vi "Editor.vi"() -> ()   [LabVIEW 2010]
uses:
  Components/Components.lvlib
panel:
  out "Current File":path caption="selected path"
  in  "Save As":bool
  in  "Refresh":bool
  in  "Update":bool
  out "Frame Size":u16=8
  in  "Frames":cluster{"Time":u32, "Powers":i16[]}[](array[cluster]) caption="Frame"
  out "Header":string
  in  "Number Of Motors":u8=2
  in  "Storage Size":enum8{"I8", "I16"}(ring)=enum."I16"
  out "File":refnum<file>
  in  "Writing?":bool
  in  "Cancel":bool
  in  "Open":bool
  in  "New":bool
  out "Binary Out":string
  in  "Save":bool
  # "4BC Editor"
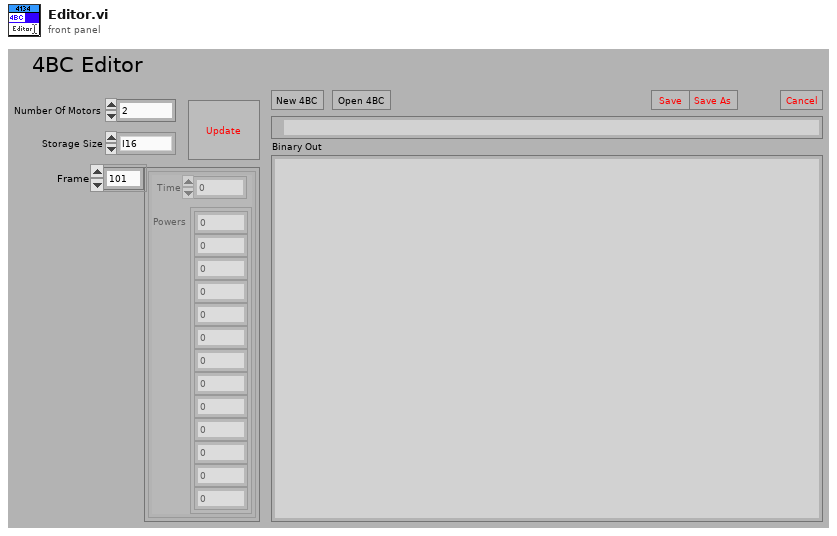
[diagram p1: front panel]
types:
  T1 = enum16{"open", "replace", "create", "open or create", "replace or create", "replace or create with confirmation"}
  T2 = enum16{"big-endian, network order", "native, host order", "little-endian"}
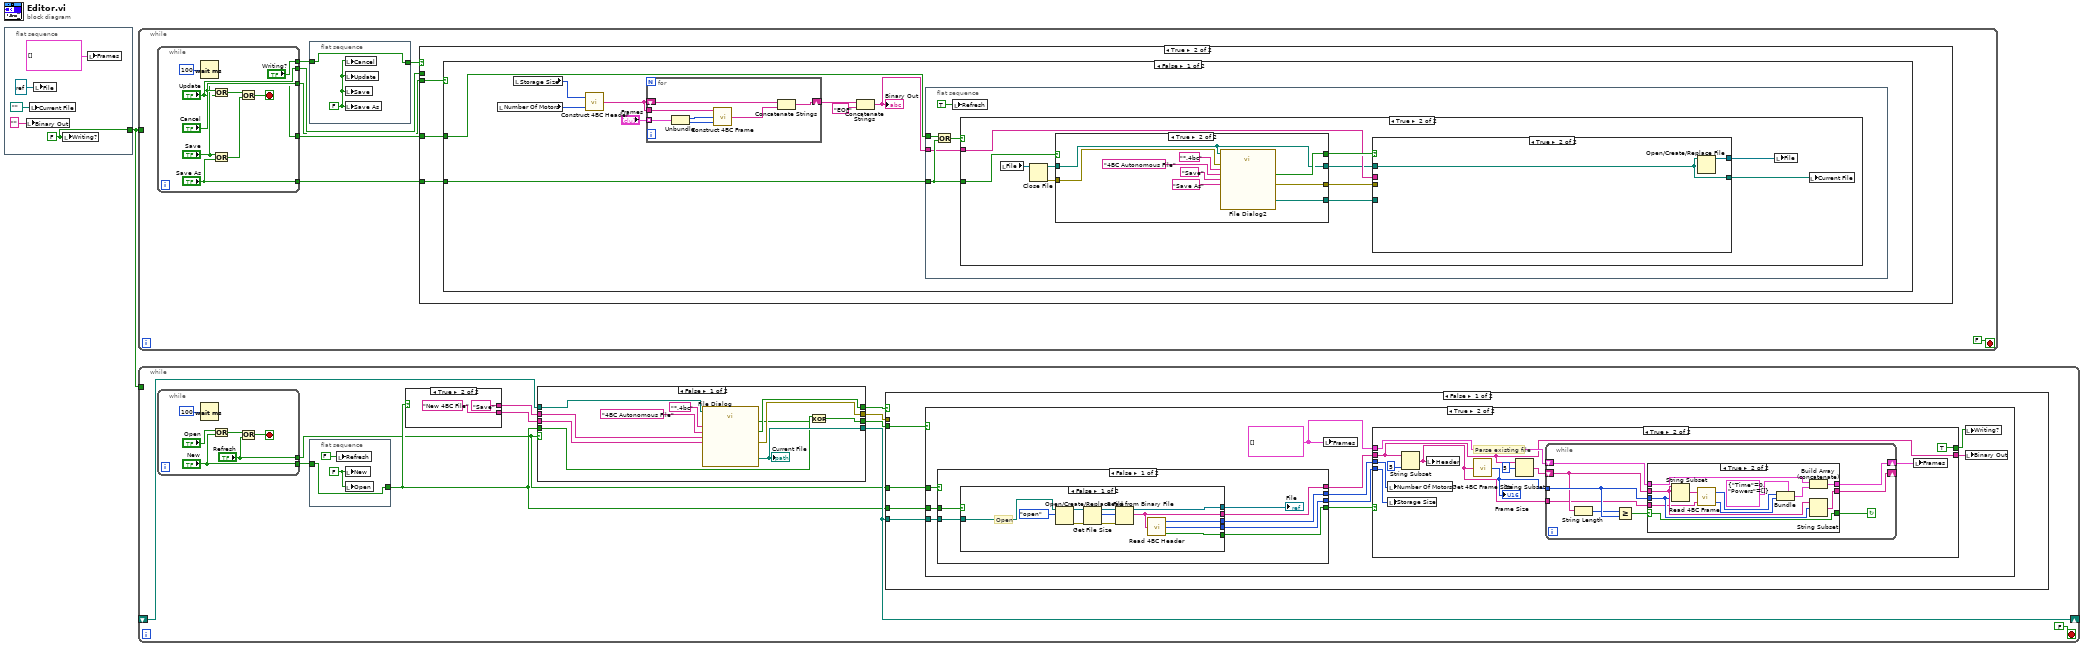
[diagram p0: block diagram]
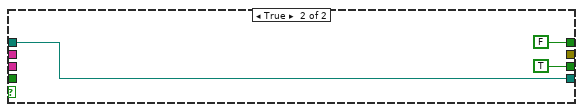
[diagram p2: hidden frame]
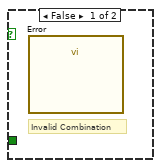
[diagram p3: hidden frame]
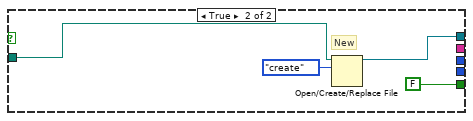
[diagram p4: hidden frame]
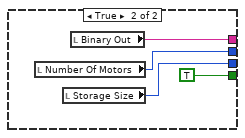
[diagram p5: hidden frame]
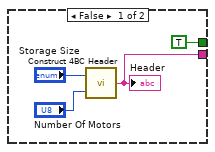
[diagram p6: hidden frame]
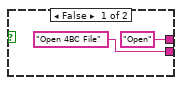
[diagram p9: hidden frame]
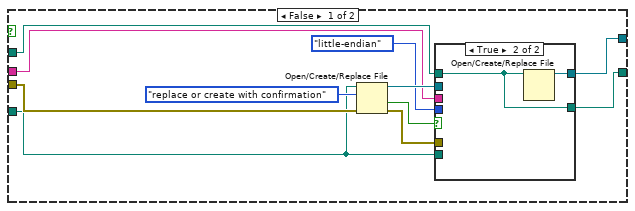
[diagram p12: hidden frame]
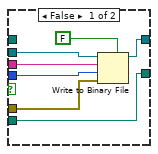
[diagram p13: hidden frame]
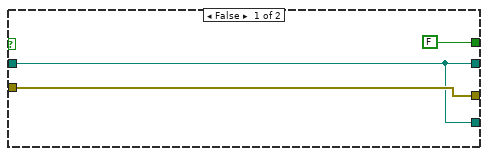
[diagram p14: hidden frame]
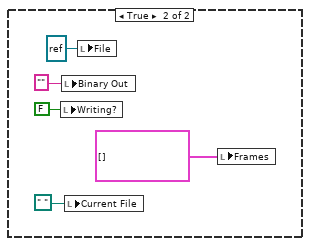
[diagram p15: hidden frame]
diagram:
  n1 = flat-sequence {
    tunnel: [w6] -> w1
    frame #0 {
      w6 = FALSE ("Writing?")
      n2 = local write "Binary Out"("" ("Binary Out")) -> ()
      n3 = local write "Current File"(path "" ("Current File")) -> ()
      n4 = local write "File"(refnum<file> refnum ("File")) -> ()
      n5 = local write "Writing?"(w6) -> ()
      n6 = local write "Frames"(cluster{"Time":u32, "Powers":i16[]}[] [] ("Frames")) -> ()
    }
  }
  n7 = while {
    tunnel: w1 -> [_]
    stop <- FALSE stop-if-true
    n8 = while {
      tunnel: ["Writing?"] -> w10
      tunnel: ["Save"] -> w11
      tunnel: ["Update"] -> w12
      tunnel: ["Cancel"] -> w8
      tunnel: ["Save As"] -> w7
      stop <- w97 stop-if-true
      n9 = Wait (ms)(milliseconds to wait=u32 100) -> ()  [unwired: 1 out]
      n10 = Or(x="Cancel", y="Update") -> (x .or. y?=w93:bool)
      n11 = Or(x="Save", y="Save As") -> (x .or. y?=w94:bool)
      n12 = Or(x=w93, y=w94) -> (x .or. y?=w97:bool)
    }
    n13 = flat-sequence {
      tunnel: w10 -> [w15]
      tunnel: [w15] -> w9
      frame #0 {
        w14 = FALSE ("Cancel")
        n14 = local write "Cancel"(w14) -> ()
        n15 = local write "Update"(w14) -> ()
        n16 = local write "Save"(w14) -> ()
        n17 = local write "Save As"(w14) -> ()
      }
    }
    n18 = case shown="True" w9 {
      tunnel: w12 -> [_ _]
      tunnel: w11 -> [_ w17]
      tunnel: w8 -> [_ w18]
      tunnel: w7 -> [_ w16]
      frame False {
      }
      frame True {
        n19 = case shown="False" w18 {
          tunnel: w17 -> [w19 _]
          tunnel: w16 -> [w20 _]
          frame False {
            n20 = local read "Number Of Motors"() -> (w26:u8)
            n21 = local read "Storage Size"() -> (w27:enum8{"I8", "I16"})
            n22 = call "Construct 4BC Header.vi"("Number Of Motors"=w26, "Storage Size"=w27) -> ("Header"=w24:string)
            n23 = for {
              shift-right: [w78] -> w23
              shift-left: w24 -> [w79]
              tunnel: "Frames" -> [w84] mode=indexing
              tunnel: w24 -> [w81]
              n24 = Unbundle(w84) -> ("Time"=w83:u32, "Powers"=w82:i16[])
              n25 = call "Construct 4BC Frame.vi"("Array"=w82, "Time"=w83, "Header"=w81) -> ("Frame"=w80:string)  [unwired: 1 in]
              n26 = Concatenate Strings(w79, w80) -> (w78:string)
            }
            n27 = Concatenate Strings(w23, "EOF" ("string")) -> (w21:string)
            "Binary Out" <- w21
            n28 = flat-sequence {
              tunnel: w21 -> [w28]
              tunnel: w20 -> [w30]
              tunnel: w19 -> [w29]
              frame #0 {
                n29 = Or(x=w29, y=w30) -> (x .or. y?=w31:bool)
                n30 = local write "Refresh"(TRUE ("Refresh")) -> ()
                n31 = case shown="True" w31 {
                  tunnel: w30 -> [_ w42]
                  tunnel: w28 -> [_ w36]
                  frame False {
                  }
                  frame True {
                    n32 = local read "File"() -> (w43:refnum<file>)
                    n33 = Close File(refnum=w43) -> (path=w41:path, error out=w40:errorcluster)  [unwired: 1 in]
                    n34 = case shown="True" w42 {
                      tunnel: w41 -> [w66 w69]
                      tunnel: w40 -> [w68 w77]
                      tunnel: [w68 w72] -> w39
                      tunnel: [w66 w71] -> w38
                      tunnel: [FALSE ("cancelled") w70] -> w37
                      tunnel: [w66 w69] -> w35
                      frame False {
                      }
                      frame True {
                        n35 = call "File Dialog2"("start path"=w69, "prompt"="Save As", "button label"="Save", "error in"=w77, "pattern (all files)"="*.4bc", "pattern label"="4BC Autonomous File") -> ("selected path"=w71:path, "cancelled"=w70:bool, "error out"=w72:errorcluster)  [unwired: 6 in, 1 out]
                      }
                    }
                    n36 = case shown="True" w37 {
                      tunnel: w39 -> [w53 _]
                      tunnel: w38 -> [w47 _]
                      tunnel: w36 -> [w51 _]
                      tunnel: w35 -> [w46 w64]
                      tunnel: [w45 w65] -> w34
                      tunnel: [w44 w64] -> w33
                      frame False {
                        n37 = Open/Create/Replace File(file path (use dialog)=w47, error in=w53, operation (0:open)=T1."replace or create with confirmation") -> (refnum out=w54:refnum<file>, cancelled=w48:bool, error out=w49:errorcluster)  [unwired: 3 in]
                        n38 = case shown="True" w48 {
                          tunnel: w54 -> [w61 _]
                          tunnel: T2."little-endian" ("byte order (0:big-endian, network order)") -> [w59 _]
                          tunnel: w51 -> [w58 _]
                          tunnel: w49 -> [w57 _]
                          tunnel: w47 -> [w55 _]
                          tunnel: [w56 w63] -> w45
                          tunnel: [w55 w62] -> w44
                          tunnel: w46 -> [_ w62]
                          frame False {
                            n39 = Write to Binary File(file (use dialog)=w61, data=w58, error in=w57, 5:FALSE ("prepend array or string size? (T)"), 9:w59) -> (refnum out=w56:refnum<file>)  [unwired: 1 in, 2 out]
                          }
                          frame True {
                            n40 = Open/Create/Replace File(file path (use dialog)=w62) -> (refnum out=w63:refnum<file>)  [unwired: 5 in, 2 out]
                          }
                        }
                      }
                      frame True {
                        n41 = Open/Create/Replace File(file path (use dialog)=w64) -> (refnum out=w65:refnum<file>)  [unwired: 5 in, 2 out]
                      }
                    }
                    n42 = local write "File"(w34) -> ()
                    n43 = local write "Current File"(w33) -> ()
                  }
                }
              }
            }
          }
          frame True {
            n44 = local write "Writing?"(FALSE ("Writing?")) -> ()
            n45 = local write "Binary Out"("" ("Binary Out")) -> ()
            n46 = local write "Current File"(path " " ("Current File")) -> ()
            n47 = local write "File"(refnum<file> refnum ("File")) -> ()
            n48 = local write "Frames"(cluster{"Time":u32, "Powers":i16[]}[] [] ("Frames")) -> ()
          }
        }
      }
    }
  }
  n49 = while {
    shift-right: [w104] -> _
    shift-left: _ -> [w106]
    tunnel: w1 -> [_]
    stop <- FALSE stop-if-true
    n50 = while {
      tunnel: ["New"] -> w105
      tunnel: ["Refresh"] -> w99
      stop <- w212 stop-if-true
      n51 = Wait (ms)(milliseconds to wait=u32 100) -> ()  [unwired: 1 out]
      n52 = Or(x="Open", y="New") -> (x .or. y?=w213:bool)
      n53 = Or(x=w213, y="Refresh") -> (x .or. y?=w212:bool)
    }
    n54 = flat-sequence {
      tunnel: w105 -> [w205]
      tunnel: [w205] -> w100
      frame #0 {
        w206 = FALSE ("New")
        n55 = local write "Refresh"(FALSE ("Refresh")) -> ()
        n56 = local write "New"(w206) -> ()
        n57 = local write "Open"(w206) -> ()
      }
    }
    n58 = case shown="True" w100 {
      tunnel: ["Open" "Save"] -> w107
      tunnel: ["Open 4BC File" "New 4BC File"] -> w108
      frame False {
      }
      frame True {
      }
    }
    n59 = case shown="False" w99 {
      tunnel: w108 -> [w118 _]
      tunnel: w107 -> [w117 _]
      tunnel: w106 -> [w116 w121]
      tunnel: [w115 w121] -> w104
      tunnel: [w114 FALSE ("cancelled")] -> w103
      tunnel: [w110 TRUE] -> w101
      tunnel: [w113 _] -> w102
      tunnel: w100 -> [w112 _]
      frame False {
        n60 = call "File Dialog"("start path"=w116, "prompt"=w118, "button label"=w117, "pattern (all files)"="*.4bc", "pattern label"="4BC Autonomous File") -> ("selected path"=w115:path, "exists"=w111:bool, "cancelled"=w114:bool, "error out"=w113:errorcluster)  [unwired: 7 in]
        "Current File" <- w115
        n61 = Exclusive Or(1:w111, 2:w112) -> (0:w110:bool)
      }
      frame True {
      }
    }
    n62 = case shown="False" w103 {
      tunnel: w104 -> [w125 _]
      tunnel: w101 -> [w127 _]
      tunnel: w100 -> [w126 _]
      tunnel: w102 -> [_ _]
      tunnel: w99 -> [w124 _]
      frame False {
        n63 = case shown="True" w127 {
          tunnel: w126 -> [_ w137]
          tunnel: w125 -> [_ w136]
          tunnel: w124 -> [_ w128]
          frame False {
            # "Invalid Combination"
            n64 = call "Error"() -> ()  [unwired: 18 in, 2 out]
          }
          frame True {
            w130 = cluster{"Time":u32, "Powers":i16[]}[] [] ("Frames 2")
            n65 = case shown="False" w128 {
              tunnel: w137 -> [w144 _]
              tunnel: w136 -> [w143 _]
              tunnel: [w141 TRUE ("Valid?")] -> w135
              tunnel: [w140 w163] -> w134
              tunnel: [w139 w161] -> w133
              tunnel: [w138 w162] -> w132
              frame False {
                n66 = case shown="False" w144 {
                  tunnel: w143 -> [w155 w159]
                  tunnel: [w156 w158] -> w142
                  tunnel: [w145 _] -> w140
                  tunnel: [w148 FALSE] -> w141
                  tunnel: [w147 _] -> w139
                  tunnel: [w146 _] -> w138
                  frame False {
                    # "Open"
                    n67 = Open/Create/Replace File(file path (use dialog)=w155, operation (0:open)=T1."open") -> (refnum out=w152:refnum<file>, error out=w150:errorcluster)  [unwired: 4 in, 1 out]
                    n68 = Get File Size(file=w152, error in=w150) -> (refnum out=w151:refnum<file>, size (in bytes)=w153:i64, 0:w149:errorcluster)
                    n69 = Read from Binary File(8:w149, 10:w153, 11:w151) -> (2:w145:string, 3:w156:refnum<file>)  [unwired: 3 in, 2 out]
                    n70 = call "Read 4BC Header.vi"("Header"=w145) -> ("Valid?"=w148:bool, "Storage Size"=w147:enum8{"I8", "I16"}, "Number Of Motors"=w146:u8)
                  }
                  frame True {
                    # "New"
                    n71 = Open/Create/Replace File(file path (use dialog)=w159, operation (0:open)=T1."create") -> (refnum out=w158:refnum<file>)  [unwired: 4 in, 2 out]
                  }
                }
                "File" <- w142
              }
              frame True {
                n72 = local read "Number Of Motors"() -> (w162:u8)
                n73 = local read "Storage Size"() -> (w161:enum8{"I8", "I16"})
                n74 = local read "Binary Out"() -> (w163:string)
              }
            }
            n75 = local write "Frames"(w130) -> ()
            n76 = case shown="True" w135 {
              tunnel: w134 -> [_ w171]
              tunnel: w133 -> [_ w179]
              tunnel: w132 -> [_ w178]
              tunnel: [w166 w171] -> w131
              tunnel: w130 -> [_ w174]
              tunnel: [TRUE ("Writing?") TRUE ("Writing?")] -> w129
              frame False {
                n77 = call "Construct 4BC Header.vi"("Number Of Motors"="Number Of Motors", "Storage Size"="Storage Size") -> ("Header"=w166:string)
                "Header" <- w166
              }
              frame True {
                # "Parse existing file"
                n78 = local write "Number Of Motors"(w178) -> ()
                n79 = local write "Storage Size"(w179) -> ()
                n80 = String Subset(string=w171, length (rest)=5 ("length (rest)")) -> (substring=w172:string)  [unwired: 1 in]
                n81 = local write "Header"(w172) -> ()
                n82 = call "Get 4BC Frame Size.vi"("Header"=w172) -> ("Frame Size"=w169:u16)
                "Frame Size" <- w169
                n83 = String Subset(string=w171, offset (0)=5) -> (substring=w176:string)  [unwired: 1 in]
                n84 = while {
                  shift-right: [w180] -> _
                  shift-left: w176 -> [w185]
                  tunnel: w169 -> [w187]
                  shift-right: [w181] -> w173
                  shift-left: w174 -> [w182]
                  tunnel: w172 -> [w183]
                  stop <- w188 continue-if-true
                  n85 = String Length(string=w185) -> (length=w186:i32)
                  n86 = Greater Or Equal?(x=w186, y=w187) -> (x >= y?=w184:bool)
                  n87 = case shown="True" w184 {
                    selector: w184 -> [w191 w203]
                    tunnel: w185 -> [w189 w196]
                    tunnel: w187 -> [_ w194]
                    tunnel: [w191 w203] -> w188
                    tunnel: w183 -> [_ w192]
                    tunnel: w182 -> [w190 w202]
                    tunnel: [w190 w197] -> w181
                    tunnel: [w189 w195] -> w180
                    frame False {
                    }
                    frame True {
                      n88 = String Subset(string=w196, length (rest)=w194) -> (substring=w193:string)  [unwired: 1 in]
                      n89 = call "Read 4BC Frame.vi"("Header"=w192, "Frame"=w193) -> ("Array"=w199:i16[], "Time"=w200:u32)
                      n90 = Bundle(cluster=cluster{"Time":u32, "Powers":i16[]} {"Time"=0, "Powers"=[]} ("Frame"), "Time"=w200, "Powers"=w199) -> (w198:cluster{"Time":u32, "Powers":i16[]})
                      n91 = Build Array (concatenate)(w202, w198) -> (w197:cluster{"Time":u32, "Powers":i16[]}[])
                      n92 = String Subset(string=w196, offset (0)=w194) -> (substring=w195:string)  [unwired: 1 in]
                    }
                  }
                }
                n93 = local write "Frames"(w173) -> ()
              }
            }
            n94 = local write "Writing?"(w129) -> ()
            n95 = local write "Binary Out"(w131) -> ()
          }
        }
      }
      frame True {
        # "Canceled"
      }
    }
  }
